vi "Validate Measurement Configuration.vi"(8 "error in":errorcluster, 11 "Measurement Configuration In":T1={"TDMS File Location"="", "Run Action"="Create/Replace Wfm Group", "Wfm Group Name"="Wfm1", "Channel Names"=[], "Waveforms Summary JSON"=[]}) -> (0 "error out":errorcluster, 3 "Measurement Configuration Out":T1)   [LabVIEW 2025, in "TDMS Waveform Creator.lvclass"]
uses:
  TDMS Waveform Creator.lvclass
  TDMS Waveform Creator.lvclass/TDMS Waveform Creator.ctl
  <vilib>/ErrorRing/Error Ring.xnode
  <vilib>/Utility/error.llb/Error Cluster From Error Code.vi
  Measurement Configuration.ctl
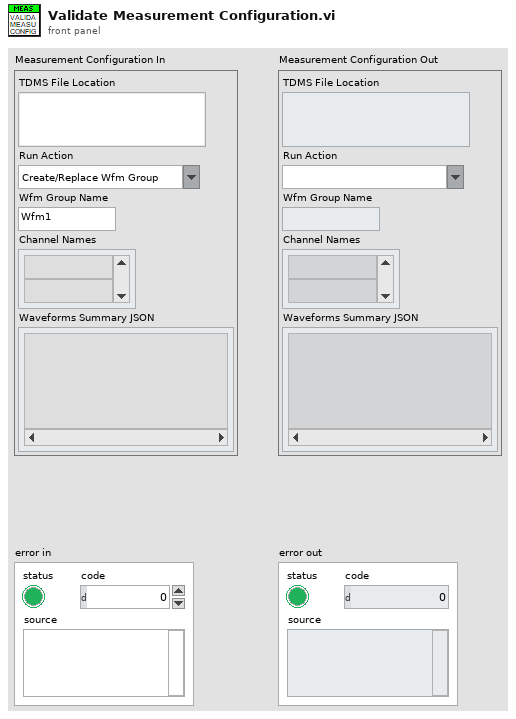
[diagram p1: front panel]
types:
  T1 = typedef "TDMS Waveform Creator.lvclass/Measurement Configuration.ctl" = cluster{"TDMS File Location":string, "Run Action":string, "Wfm Group Name":string, "Channel Names":string[], "Waveforms Summary JSON":string[]}
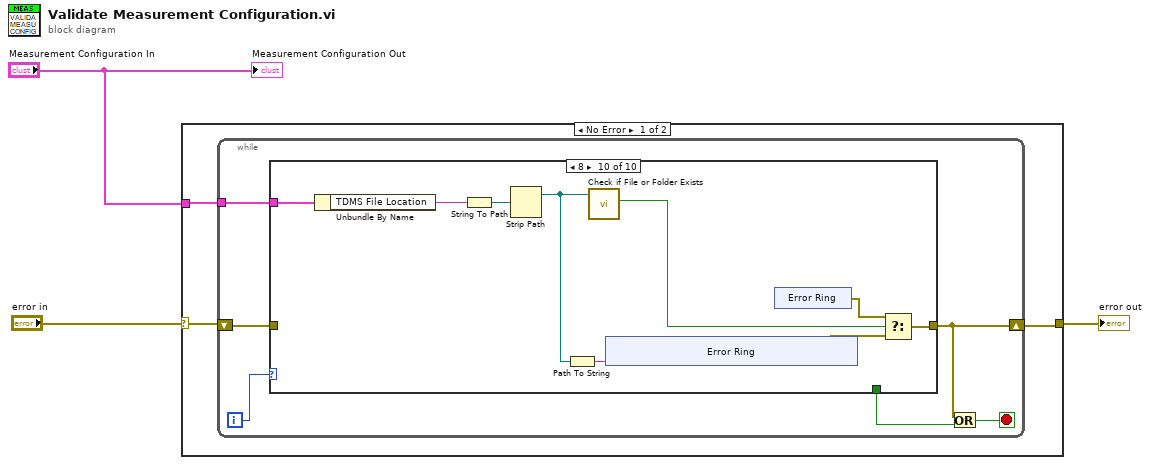
[diagram p0: block diagram]
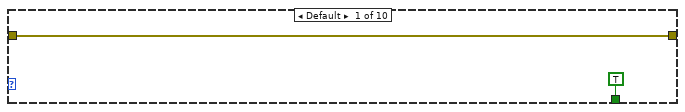
[diagram p2: hidden frame]
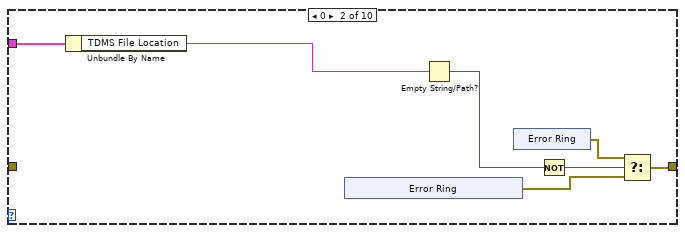
[diagram p3: hidden frame]
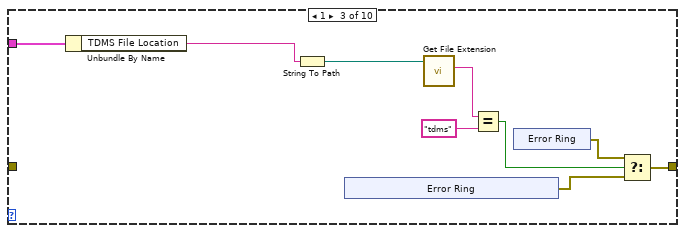
[diagram p4: hidden frame]
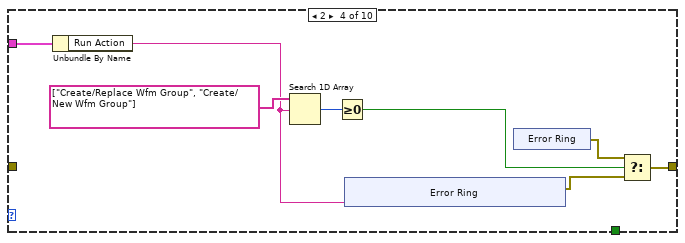
[diagram p5: hidden frame]
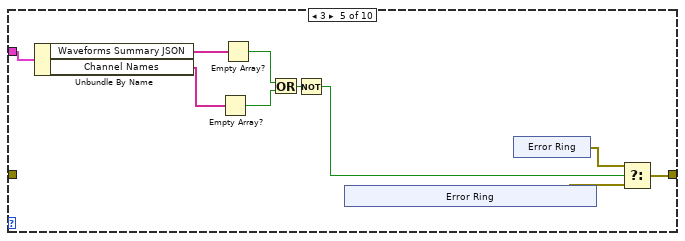
[diagram p6: hidden frame]
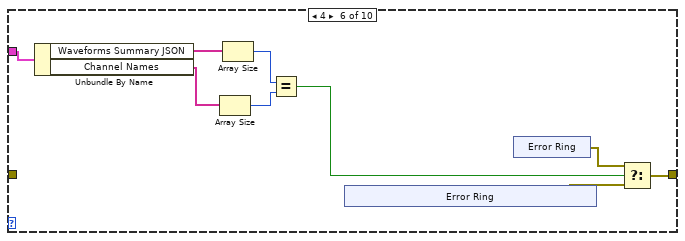
[diagram p7: hidden frame]
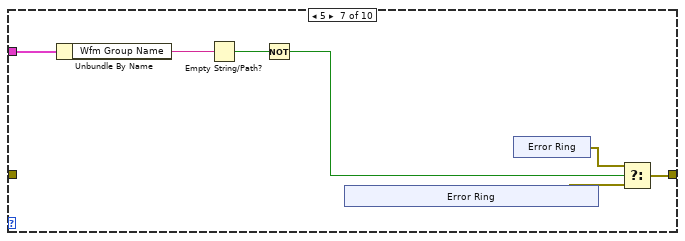
[diagram p8: hidden frame]
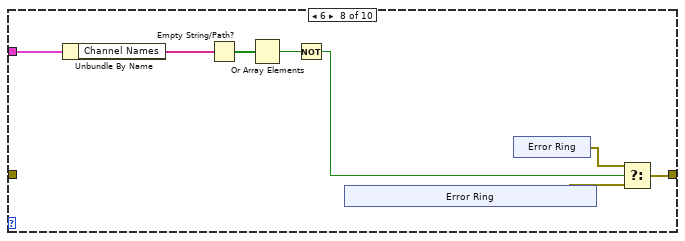
[diagram p9: hidden frame]
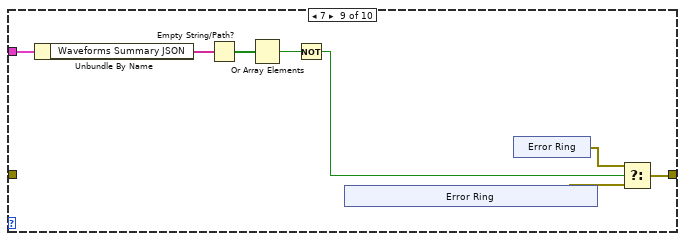
[diagram p10: hidden frame]
diagram:
  n1 = case shown="No Error" "error in" {
    selector: "error in" -> [w4 w148]
    tunnel: [w5 w148] -> w2
    tunnel: "Measurement Configuration In" -> [w6 _]
    frame No Error {
      n2 = while {
        tunnel: w6 -> [w12]
        shift-right: [w7] -> w5
        shift-left: w4 -> [w9]
        i -> [w11]
        stop <- w8 stop-if-true
        n3 = case shown="8" w11 {
          tunnel: w12 -> [_ w21 w36 w50 w68 w83 w96 w110 w124 w139]
          tunnel: [TRUE _ _ _ _ _ _ _ _ _] -> w10
          tunnel: [w13 w16 w33 w47 w65 w80 w93 w107 w121 w136] -> w7
          tunnel: w9 -> [w13 _ _ _ _ _ _ _ _ _]
          frame Default {
          }
          frame 0 {
            n4 = Unbundle By Name(w21) -> ("TDMS File Location"=w20:string)
            n5 = xnode "Error Ring"() -> ("error out"=w17:errorcluster)
            n6 = Empty String/Path?(string/path=w20) -> (empty?=w19:bool)
            n7 = xnode "Error Ring"() -> ("error out"=w18:errorcluster)
            n8 = Not(x=w19) -> (.not. x?=w15:bool)
            n9 = Select(t=w18, s=w15, f=w17) -> (s? t:f=w16:errorcluster)
          }
          frame 1 {
            n10 = Unbundle By Name(w36) -> ("TDMS File Location"=w31:string)
            n11 = String To Path(string=w31) -> (path=w32:path)
            n12 = xnode "Error Ring"() -> ("error out"=w34:errorcluster)
            n13 = call <vilib>:"Get File Extension.vi"("file"=w32) -> ("lowercase file extension"=w30:string)  [unwired: 6 in, 4 out]
            n14 = Equal?(x=w30, y="tdms") -> (x = y?=w28:bool)
            n15 = xnode "Error Ring"() -> ("error out"=w35:errorcluster)
            n16 = Select(t=w35, s=w28, f=w34) -> (s? t:f=w33:errorcluster)
          }
          frame 2 {
            n17 = Unbundle By Name(w50) -> ("Run Action"=w44:string)
            n18 = Search 1D Array(1D array=string[] ["Create/Replace Wfm Group", "Create/New Wfm Group"] ("Run Action"), element=w44) -> (index of element=w45:i32)  [unwired: 1 in]
            n19 = Greater Or Equal To 0?(x=w45) -> (x >= 0?=w43:bool)
            n20 = xnode "Error Ring"("parameter 0"=w44) -> ("error out"=w48:errorcluster)
            n21 = xnode "Error Ring"() -> ("error out"=w49:errorcluster)
            n22 = Select(t=w49, s=w43, f=w48) -> (s? t:f=w47:errorcluster)
          }
          frame 3 {
            n23 = Unbundle By Name(w68) -> ("Waveforms Summary JSON"=w63:string[], "Channel Names"=w64:string[])
            n24 = Empty Array?(array=w64) -> (empty?=w61:bool)
            n25 = Empty Array?(array=w63) -> (empty?=w62:bool)
            n26 = Or(x=w62, y=w61) -> (x .or. y?=w60:bool)
            n27 = Not(x=w60) -> (.not. x?=w59:bool)
            n28 = xnode "Error Ring"() -> ("error out"=w66:errorcluster)
            n29 = xnode "Error Ring"() -> ("error out"=w67:errorcluster)
            n30 = Select(t=w67, s=w59, f=w66) -> (s? t:f=w65:errorcluster)
          }
          frame 4 {
            n31 = Unbundle By Name(w83) -> ("Waveforms Summary JSON"=w78:string[], "Channel Names"=w79:string[])
            n32 = Array Size(array=w79) -> (size(s)=w76:i32)
            n33 = Array Size(array=w78) -> (size(s)=w77:i32)
            n34 = Equal?(x=w77, y=w76) -> (x = y?=w75:bool)
            n35 = xnode "Error Ring"() -> ("error out"=w81:errorcluster)
            n36 = xnode "Error Ring"() -> ("error out"=w82:errorcluster)
            n37 = Select(t=w82, s=w75, f=w81) -> (s? t:f=w80:errorcluster)
          }
          frame 5 {
            n38 = Unbundle By Name(w96) -> ("Wfm Group Name"=w92:string)
            n39 = Empty String/Path?(string/path=w92) -> (empty?=w91:bool)
            n40 = Not(x=w91) -> (.not. x?=w90:bool)
            n41 = xnode "Error Ring"() -> ("error out"=w94:errorcluster)
            n42 = xnode "Error Ring"() -> ("error out"=w95:errorcluster)
            n43 = Select(t=w95, s=w90, f=w94) -> (s? t:f=w93:errorcluster)
          }
          frame 6 {
            n44 = Unbundle By Name(w110) -> ("Channel Names"=w106:string[])
            n45 = Empty String/Path?(string/path=w106) -> (empty?=w105:bool[])
            n46 = Or Array Elements(Boolean array=w105) -> (logical OR=w103:bool)
            n47 = Not(x=w103) -> (.not. x?=w104:bool)
            n48 = xnode "Error Ring"() -> ("error out"=w108:errorcluster)
            n49 = xnode "Error Ring"() -> ("error out"=w109:errorcluster)
            n50 = Select(t=w109, s=w104, f=w108) -> (s? t:f=w107:errorcluster)
          }
          frame 7 {
            n51 = Unbundle By Name(w124) -> ("Waveforms Summary JSON"=w120:string[])
            n52 = Empty String/Path?(string/path=w120) -> (empty?=w119:bool[])
            n53 = Or Array Elements(Boolean array=w119) -> (logical OR=w117:bool)
            n54 = Not(x=w117) -> (.not. x?=w118:bool)
            n55 = xnode "Error Ring"() -> ("error out"=w122:errorcluster)
            n56 = xnode "Error Ring"() -> ("error out"=w123:errorcluster)
            n57 = Select(t=w123, s=w118, f=w122) -> (s? t:f=w121:errorcluster)
          }
          frame 8 {
            n58 = Unbundle By Name(w139) -> ("TDMS File Location"=w135:string)
            n59 = String To Path(string=w135) -> (path=w134:path)
            n60 = Strip Path(path=w134) -> (stripped path=w132:path)  [unwired: 1 out]
            n61 = Path To String(path=w132) -> (string=w131:string)
            n62 = call <vilib>:"Check if File or Folder Exists.vi"("path"=w132) -> ("file or folder exists?"=w133:bool)  [unwired: 8 in, 2 out]
            n63 = xnode "Error Ring"("parameter 0"=w131) -> ("error out"=w137:errorcluster)
            n64 = xnode "Error Ring"() -> ("error out"=w138:errorcluster)
            n65 = Select(t=w138, s=w133, f=w137) -> (s? t:f=w136:errorcluster)
          }
        }
        n66 = Or(x=w7, y=w10) -> (x .or. y?=w8:bool)
      }
    }
    frame Error {
    }
  }
  "error out" <- w2
  "Measurement Configuration Out" <- "Measurement Configuration In"
